vi "Trapezoidal integration.vi"(1 "dt":sgl, 2 "Input waveform":sgl[](array[numeric])) -> (0 "output value":sgl)   [LabVIEW 2010]
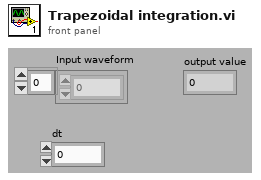
[diagram p1: front panel]
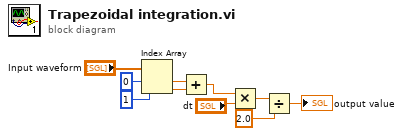
[diagram p0: block diagram]
diagram:
  n1 = Index Array(array="Input waveform", index #1=0 ("index"), index #2=1 ("index")) -> (element #1=w7:sgl, element #2=w8:sgl)
  n2 = Add(x=w7, y=w8) -> (x+y=w6:sgl)
  n3 = Multiply(x=w6, y="dt") -> (x*y=w5:sgl)
  n4 = Divide(x=w5, y=sgl 2.0) -> (x/y=→"output value":sgl)
